vi "Global_CMD_ACT_Data In.vi"() -> ()   [LabVIEW 2023, in "Template FX_ACT.lvlib"]
uses:
  Template FX_ACT.lvlib
  Cluster_CMD_ACT_Data.ctl
  ENUM_CMD_Mode Select.ctl
panel:
  in  "CMD_ACT_Tempplate Data":T1
  # "The Names of the Data items in the Global Variable MUST describe who the Single Writer is\nFor Command Globals the Commander(CMD) represents Teleop or Autonomous or other command loop.\nThe naming convention for a Command Actuator Global is:   \n\nCMD_ACT_SubSystem_Data Name\n\nExample:\nCMD_ACT_Drive_Data\nCMD_ACT_Hopper_Eject Ball"
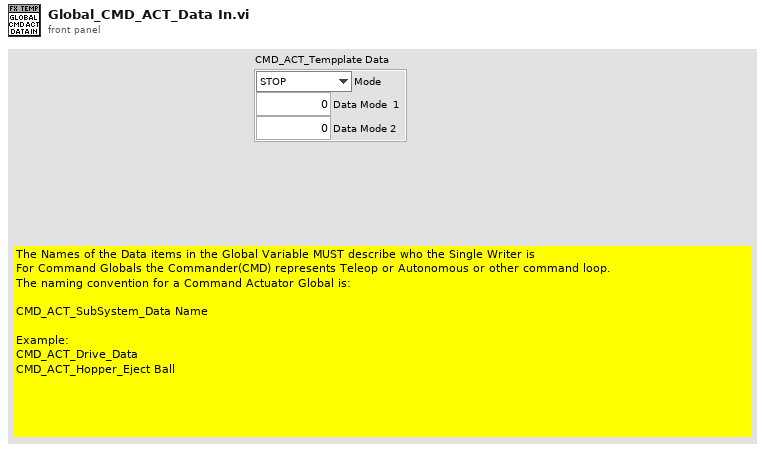
[diagram p1: front panel]
types:
  T1 = typedef "Template FX_ACT.lvlib/Cluster_CMD_ACT_Data.ctl" = cluster{"Mode":T2, "Data Mode  1":dbl, "Data Mode 2":dbl}
  T2 = typedef "Template FX_ACT.lvlib/ENUM_CMD_Mode Select.ctl" = enum16{"STOP", "Mode 1", "Mode 2"}
diagram:
